vi "Read AI_index.vi"(8 "error in (no error)":errorcluster, 11 "bronkhorst_reg in":refnum<class "bronkhorst_reg.lvclass">) -> (0 "error out":errorcluster, 2 "AI_index":i32, 3 "bronkhorst_reg out":refnum<class "bronkhorst_reg.lvclass">)   [LabVIEW 2019, in "bronkhorst_reg.lvclass"]
uses:
  bronkhorst_reg.lvclass
  bronkhorst_reg.lvclass/bronkhorst_reg.ctl
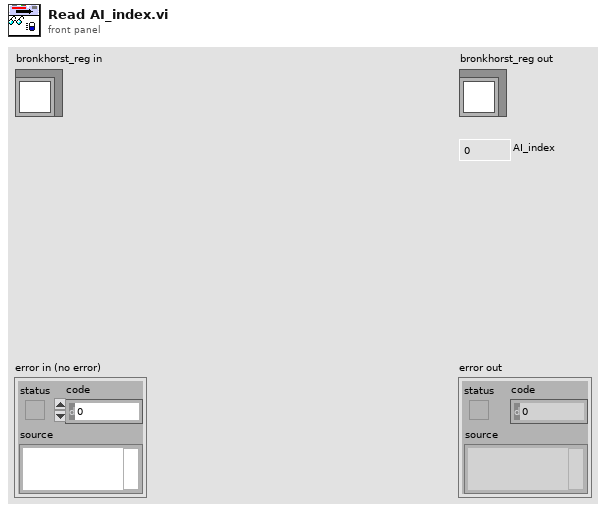
[diagram p1: front panel]
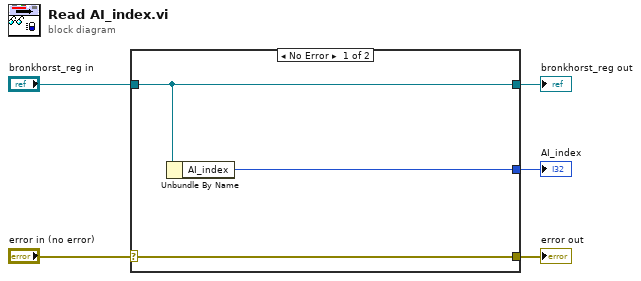
[diagram p0: block diagram]
diagram:
  n1 = case shown="No Error" "error in (no error)" {
    selector: "error in (no error)" -> [w8 w9]
    tunnel: [w8 w9] -> w4
    tunnel: [w7 w10] -> w2
    tunnel: "bronkhorst_reg in" -> [w7 w10]
    tunnel: [w6 _] -> w1
    frame No Error {
      n2 = Unbundle By Name(w7) -> ("AI_index"=w6:i32)
    }
    frame Error {
    }
  }
  "error out" <- w4
  "bronkhorst_reg out" <- w2
  "AI_index" <- w1
